vi "Offline_Analysis_SWSVM_newSelectionMethod_in_분석기.vi"(0 "LDA_matrix":path caption="LDA_matrix.txt", 1 "Target":path, 2 "Nontarget":path, 3 "in_matrix":path caption="in", 5 "svm_model_file":string, 7 "Target_order.txt":path, 9 "mius_flash_order":path, 11 "Brain":path, 12 "피험자이름":string="홍길동", 13 "Save_path":string) -> ()   [LabVIEW 2014]
uses:
  <vilib>/Utility/file.llb/Read From Spreadsheet File (DBL).vi
  <vilib>/Analysis/Matrix/Numeric/Conversions/Array To Matrix - RA2.vi
  <vilib>/Analysis/Matrix/Numeric/Conversions/Array To Matrix - RA.vi
  <vilib>/Utility/file.llb/Read From Spreadsheet File (I64).vi
  <vilib>/Utility/file.llb/Write To Spreadsheet File (DBL).vi
  <vilib>/Utility/file.llb/Write To Spreadsheet File (I64).vi
  <vilib>/Utility/file.llb/Write To Spreadsheet File (string).vi
  <vilib>/Analysis/Matrix/NI_Matrix.lvlib
panel:
  out "ACC":i16
  out "Target_order":i64[](array[numeric])
  out "Selected_Target":i32[](array[numeric])
  out "Accuracy":i16[](array[numeric])
  out "error out":errorcluster
  in  "Random_num":i32=6
  in  "Flash_Repeat":i32=20
  in  "Frame_Length":i32=10
  in  "Sampling_Rate":dbl=250.0
  # "ERP_Parameter안씀. LDA바로 집어넣으면 됨"
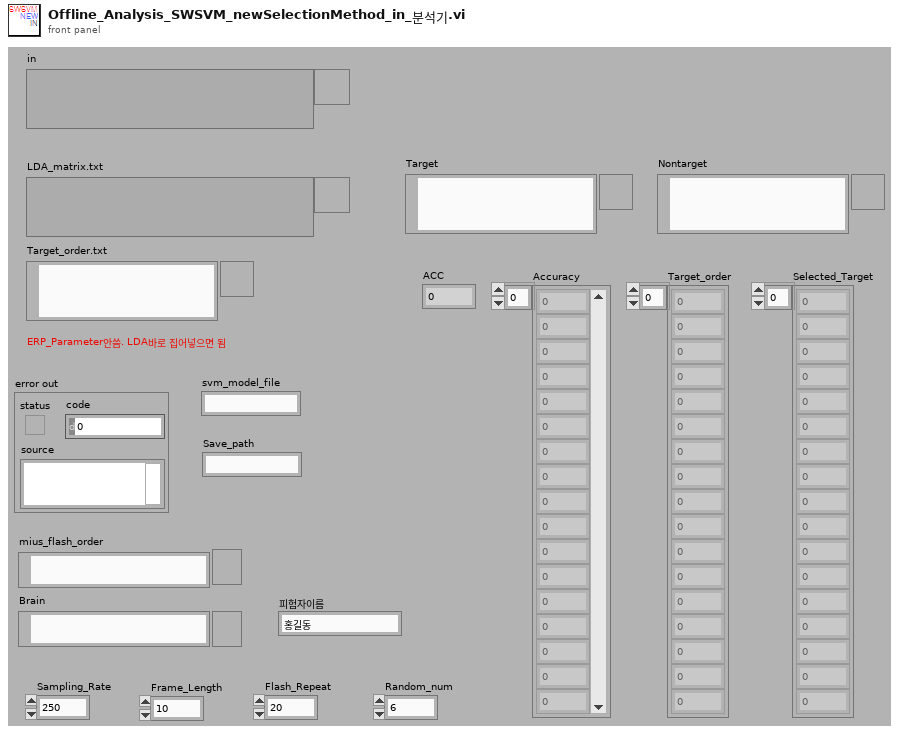
[diagram p1: front panel]
types:
  T1 = typedef "NI_Matrix.lvlib/RealMatrix.ctl" = dbl[][]
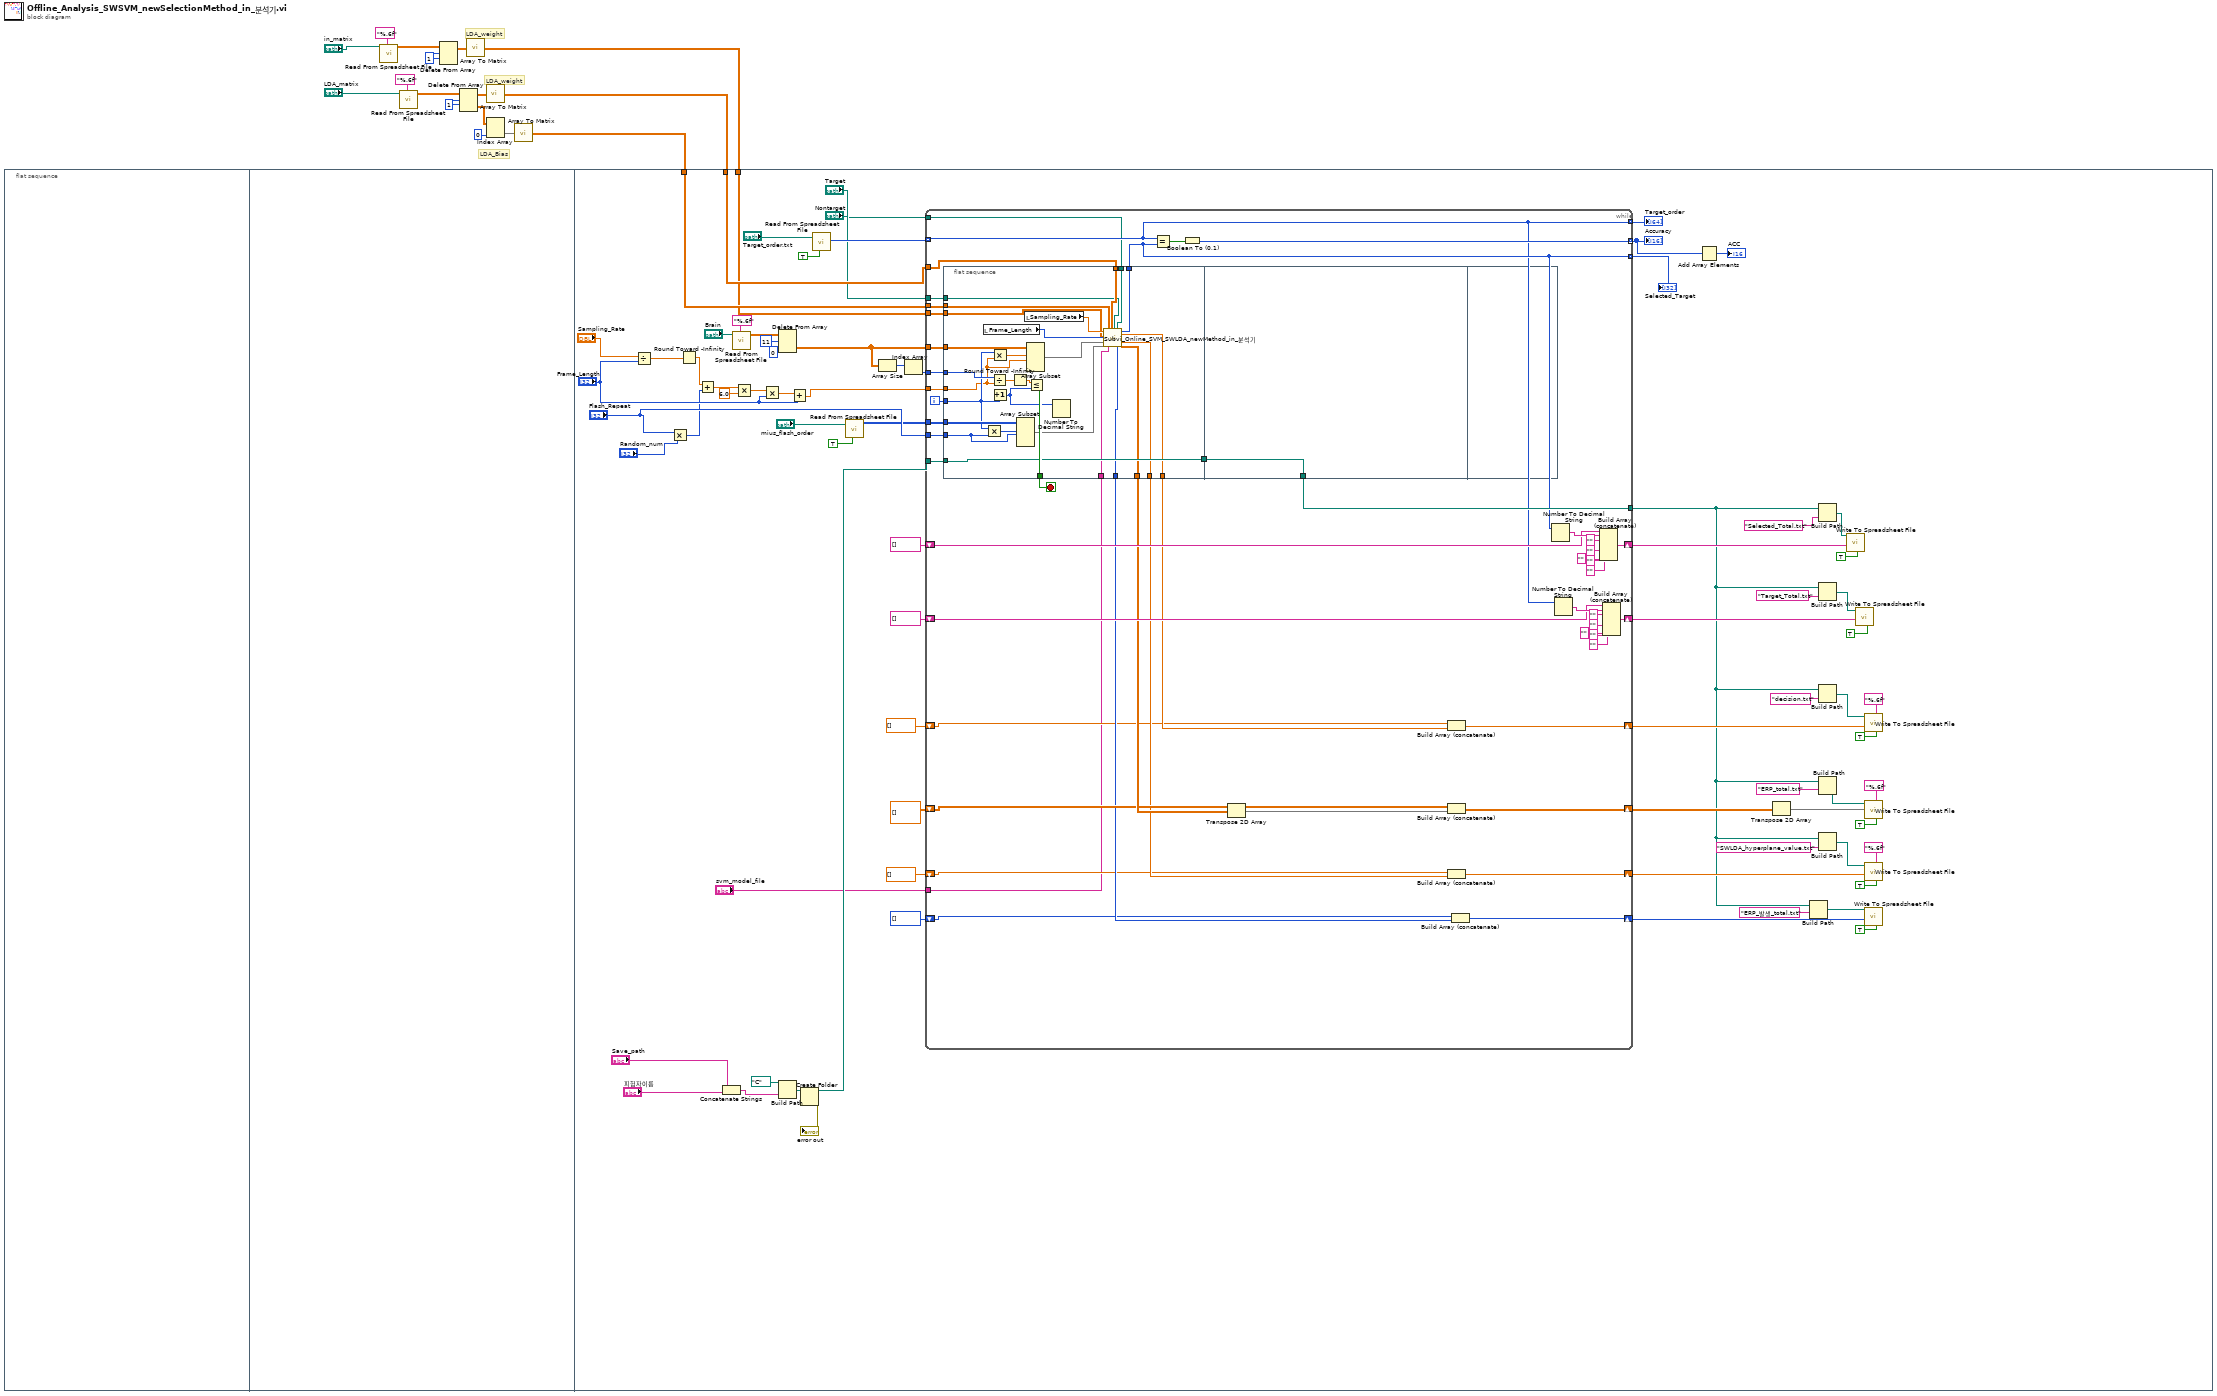
[diagram p0: block diagram]
diagram:
  w4 = 1 ("인덱스 (행)")
  w11 = 1 ("인덱스 (행)")
  # "LDA_weight"
  # "LDA_Bias"
  # "LDA_weight"
  n1 = flat-sequence {
    tunnel: w8 -> [w38]
    tunnel: w7 -> [w37]
    tunnel: w1 -> [w17]
    frame #0 {
    }
    frame #1 {
    }
    frame #2 {
      n2 = Divide(x="Sampling_Rate", y="Frame_Length") -> (x/y=w78:dbl)
      n3 = Multiply(x="Flash_Repeat", y="Random_num") -> (x*y=w81:i32)
      n4 = Round Toward -Infinity(1:w78) -> (0:w80:dbl)
      n5 = Add(x=w80, y=w81) -> (x+y=w83:dbl)
      n6 = Concatenate Strings("Save_path", "피험자이름") -> (w22:string)
      n7 = call-poly <vilib>:"Read From Spreadsheet File.vi"("format (%.3f)"="%.6f", "file path (dialog if empty)"="Brain") -> ("all rows"=w72:dbl[][])  [unwired: 5 in, 4 out]
      n8 = Multiply(x=w83, y=6.0) -> (x*y=w85:dbl)
      n9 = Multiply(x=w85, y="Frame_Length") -> (x*y=w87:dbl)
      n10 = Build Path(base path=path "C:/" ("path"), name or relative path=w22) -> (appended path=w90:path)
      n11 = Delete From Array(array=w72, length=11 ("길이"), index (col)=0 ("비활성화된 인덱스 (열)")) -> (deleted portion=w36:dbl[][])  [unwired: 1 in, 1 out]
      n12 = Add(x=w87, y="Frame_Length") -> (x+y=w88:dbl)
      n13 = Create Folder(path (use dialog)=w90) -> (created path=w92:path, error out=→"error out":errorcluster)  [unwired: 2 in, 1 out]
      n14 = call-poly <vilib>:"Read From Spreadsheet File.vi"("transpose (no:F)"=TRUE, "file path (dialog if empty)"="Target_order.txt") -> ("first row"=w66:i64[])  [unwired: 5 in, 4 out]
      n15 = call-poly <vilib>:"Read From Spreadsheet File.vi"("transpose (no:F)"=TRUE, "file path (dialog if empty)"="mius_flash_order") -> ("all rows"=w74:i64[][])  [unwired: 5 in, 4 out]
      n16 = Array Size(array=w36) -> (size(s)=w75:i32[])
      n17 = Index Array(array=w75) -> (element=w76:i32)  [unwired: 1 in]
      n18 = while {
        tunnel: w37 -> [w143]
        tunnel: w38 -> [w142]
        tunnel: w36 -> [w140]
        tunnel: w74 -> [w139]
        tunnel: w76 -> [w141]
        tunnel: w88 -> [w137]
        tunnel: "Flash_Repeat" -> [w138]
        tunnel: w92 -> [w136]
        tunnel: w66 -> [w114] mode=indexing
        tunnel: [w133] -> w58 mode=indexing
        tunnel: [w114] -> w63 mode=indexing
        tunnel: [w115] -> w64 mode=indexing
        tunnel: [w130] -> w24
        shift-right: [w117] -> w52
        shift-left: string[] [] -> [w116]
        shift-right: [w113] -> w51
        shift-left: string[] [] -> [w112]
        shift-right: [w109] -> w46
        shift-left: dbl[][] [] -> [w108]
        shift-right: [w106] -> w39
        shift-left: i16[] [] -> [w105]
        shift-right: [w103] -> w32
        shift-left: dbl[] [] -> [w102]
        shift-right: [w100] -> w25
        shift-left: dbl[] [] -> [w99]
        tunnel: "svm_model_file" -> [w98]
        tunnel: "Target" -> [w97]
        tunnel: "Nontarget" -> [w96]
        tunnel: w17 -> [w95]
        i -> [w132]
        stop <- w131 stop-if-true
        n19 = flat-sequence {
          tunnel: w143 -> [w171]
          tunnel: w142 -> [w170]
          tunnel: w141 -> [w169]
          tunnel: [w168] -> w131
          tunnel: w140 -> [w167]
          tunnel: w139 -> [w164]
          tunnel: w138 -> [w162]
          tunnel: w132 -> [w161]
          tunnel: w137 -> [w160]
          tunnel: w136 -> [w153]
          tunnel: [w153] -> w135
          tunnel: [w154] -> w115
          tunnel: [w152] -> w111
          tunnel: [w151] -> w107
          tunnel: [w149] -> w104
          tunnel: [w148] -> w101
          tunnel: w98 -> [w147]
          tunnel: w97 -> [w146]
          tunnel: w96 -> [w145]
          tunnel: w95 -> [w144]
          tunnel: w135 -> [w172]
          tunnel: [w172] -> w130
          frame #0 {
            n20 = local read "Frame_Length"() -> (w156:i32)
            n21 = Multiply(x=w161, y=w162) -> (x*y=w163:i32)
            n22 = Divide(x=w169, y=w160) -> (x/y=w159:dbl)
            n23 = Multiply(x=w161, y=w160) -> (x*y=w166:dbl)
            n24 = Increment(x=w161) -> (x+1=w155:i32)
            n25 = Round Toward -Infinity(1:w159) -> (0:w158:dbl)
            n26 = Array Subset(array=w164, index (row)=w163, length (row)=w162) -> (w150:i64[][])  [unwired: 2 in]
            n27 = local read "Sampling_Rate"() -> (w157:dbl)
            n28 = Array Subset(array=w167, index (row)=w166, length (row)=w160) -> (w165:dbl[][])  [unwired: 2 in]
            n29 = Less Or Equal?(x=w158, y=w155) -> (x <= y?=w168:bool)
            n30 = Number To Decimal String(number=w155) -> ()  [unwired: 1 in, 1 out]
            n31 = call "Subvi_Online_SVM_SWLDA_newMethod_in_분석기.vi"("rate"=w157, "samples per channel"=w156, "in"=w144, "Brain_data_source"=w165, "Target_Flash_Order"=w150, "Value"=w171, "svm_model_file"=w147, "Matrix"=w170, "Target"=w146, "Nontarget"=w145) -> ("EPR_발생_total"=w151:i16[], "output-0~8"=w154:i32, "decision"=w148:dbl[], "SWLDA"=w149:dbl[], "ERP_Parameters"=w152:dbl[][])  [unwired: 5 in]
          }
          frame #1 {
          }
          frame #2 {
          }
        }
        n32 = Equal?(x=w114, y=w115) -> (x = y?=w134:bool)
        n33 = Boolean To (0,1)(Boolean=w134) -> (0, 1=w133:i16)
        n34 = Transpose 2D Array(2D array=w111) -> (transposed array=w110:dbl[][])
        n35 = Build Array (concatenate)(w99, w101) -> (w100:dbl[])
        n36 = Build Array (concatenate)(w108, w110) -> (w109:dbl[][])
        n37 = Build Array (concatenate)(w102, w104) -> (w103:dbl[])
        n38 = Build Array (concatenate)(w105, w107) -> (w106:i16[])
        n39 = Number To Decimal String(number=w115) -> (decimal integer string=w123:string)  [unwired: 1 in]
        n40 = Number To Decimal String(number=w114) -> (decimal integer string=w129:string)  [unwired: 1 in]
        n41 = Build Array (concatenate)(w116, w123, "" ("element"), "" ("element"), "" ("element"), "" ("element"), "" ("element")) -> (w117:string[])
        n42 = Build Array (concatenate)(w112, w129, "" ("element"), "" ("element"), "" ("element"), "" ("element"), "" ("element")) -> (w113:string[])
      }
      "Accuracy" <- w58
      "Selected_Target" <- w64
      "Target_order" <- w63
      n43 = Add Array Elements(numeric array=w58) -> (sum=→"ACC":i16)
      n44 = Transpose 2D Array(2D array=w46) -> (transposed array=w44:dbl[][])
      n45 = Build Path(base path=w24, name or relative path="ERP_발생_total.txt") -> (appended path=w41:path)
      n46 = Build Path(base path=w24, name or relative path="Selected_Total.txt") -> (appended path=w54:path)
      n47 = Build Path(base path=w24, name or relative path="Target_Total.txt") -> (appended path=w60:path)
      n48 = Build Path(base path=w24, name or relative path="decision.txt") -> (appended path=w26:path)
      n49 = Build Path(base path=w24, name or relative path="ERP_total.txt") -> (appended path=w47:path)
      n50 = Build Path(base path=w24, name or relative path="SWLDA_hyperplane_value.txt") -> (appended path=w34:path)
      n51 = call-poly <vilib>:"Write To Spreadsheet File.vi"("transpose? (no:F)"=TRUE, "1D data"=w52, "file path (dialog if empty)"=w54) -> ()  [unwired: 5 in, 1 out]
      n52 = call-poly <vilib>:"Write To Spreadsheet File.vi"("transpose? (no:F)"=TRUE, "1D data"=w51, "file path (dialog if empty)"=w60) -> ()  [unwired: 5 in, 1 out]
      n53 = call-poly <vilib>:"Write To Spreadsheet File.vi"("transpose? (no:F)"=TRUE, "format (%.3f)"="%.6f", "1D data"=w25, "file path (dialog if empty)"=w26) -> ()  [unwired: 4 in, 1 out]
      n54 = call-poly <vilib>:"Write To Spreadsheet File.vi"("transpose? (no:F)"=TRUE, "format (%.3f)"="%.6f", "2D data"=w44, "file path (dialog if empty)"=w47) -> ()  [unwired: 4 in, 1 out]
      n55 = call-poly <vilib>:"Write To Spreadsheet File.vi"("transpose? (no:F)"=TRUE, "format (%.3f)"="%.6f", "1D data"=w32, "file path (dialog if empty)"=w34) -> ()  [unwired: 4 in, 1 out]
      n56 = call-poly <vilib>:"Write To Spreadsheet File.vi"("transpose? (no:F)"=TRUE, "1D data"=w39, "file path (dialog if empty)"=w41) -> ()  [unwired: 5 in, 1 out]
    }
  }
  n57 = call-poly <vilib>:"Read From Spreadsheet File.vi"("format (%.3f)"="%.6f", "file path (dialog if empty)"="in_matrix") -> ("all rows"=w3:dbl[][])  [unwired: 5 in, 4 out]
  n58 = call-poly <vilib>:"Read From Spreadsheet File.vi"("format (%.3f)"="%.6f", "file path (dialog if empty)"="LDA_matrix") -> ("all rows"=w9:dbl[][])  [unwired: 5 in, 4 out]
  n59 = Delete From Array(array=w3, length=w4, index (row)=w4) -> (array with subset deleted=w5:dbl[][])  [unwired: 1 in, 1 out]
  n60 = Delete From Array(array=w9, length=w11, index (row)=w11) -> (deleted portion=w14:dbl[][], array with subset deleted=w13:dbl[][])  [unwired: 1 in]
  n61 = call-poly <vilib>:"Array To Matrix.vi"("Real 2D Array"=w5) -> ("Real Matrix"=w1:T1)
  n62 = call-poly <vilib>:"Array To Matrix.vi"("Real 2D Array"=w13) -> ("Real Matrix"=w8:T1)
  n63 = Index Array(array=w14, index (col)=0 ("인덱스")) -> (element=w12:dbl[])  [unwired: 1 in]
  n64 = call-poly <vilib>:"Array To Matrix.vi"("Real 1D Array"=w12) -> ("Real Matrix (Column Vector)"=w7:T1)
